vi "FPGA Main.vi"() -> ()   [LabVIEW 2017]
doc: "This VI will continually read single point values from 4 channels of an analog input module at a specified rate."
uses:
  <vilib>/LabVIEW Targets/FPGA/cRIO/shared/nicrio_ModuleControls/nicrio_cRIO-9205_VoltageRange.ctl
  <vilib>/LabVIEW Targets/FPGA/cRIO/shared/nicrio_ModuleControls/nicrio_cRIO-9205_TerminalMode.ctl
  <vilib>/rvi/Emulation/niFpgaGetClockAttributes.vi
  <vilib>/rvi/Emulation/niFpgaSctlEmulationGetInTimedLoop.vi
  <vilib>/rvi/Emulation/niFpgaEmulationReportErrorSimple.vi
  Instance           1 31Saved   NI 9203 Basic IO (FPGA) .vi
  <vilib>/rvi/eio/common/nirviEmuTemplateMethod_errors.vi
  <vilib>/rvi/interface/RandomDataEmulation/niFpgaRandomDataHandleErrors.vi
  <vilib>/rvi/Emulation/niFpgaCriticalErrorInLSC.vi
  <vilib>/eio/EIOMethodNode/EIOMethodNode.xnode
  <vilib>/eio/EIONode/EIONode.xnode
  <vilib>/rvi/DataTransferAndStorage/Container/XNode/niFpgaContainer.xnode
  <vilib>/rvi/interface/RandomDataEmulation/nirviRandomDataFpgaReadWriteTemplate.vi
panel:
  in  "AI Channel Settings":T3(array[cluster])=[{"Voltage Range"=enum."+/- 10V", "Terminal Mode"=enum."RSE"}, {"Voltage Range"=enum."+/- 10V", "Terminal Mode"=enum."RSE"}, {"Voltage Range"=enum."+/- 10V", "Terminal Mode"=enum."RSE"}, {"Voltage Range"=enum."+/- 10V", "Terminal Mode"=enum."RSE"}]
  out "Data FIFO Full":bool
  out "FPGA Error Out":errorcluster
  in  "Update AI Settings":bool
  in  "Loop Rate (uS)":u32
  in  "Stop":bool
  # "For instructions, and select Help>>Show Context Help and hover over the icon."
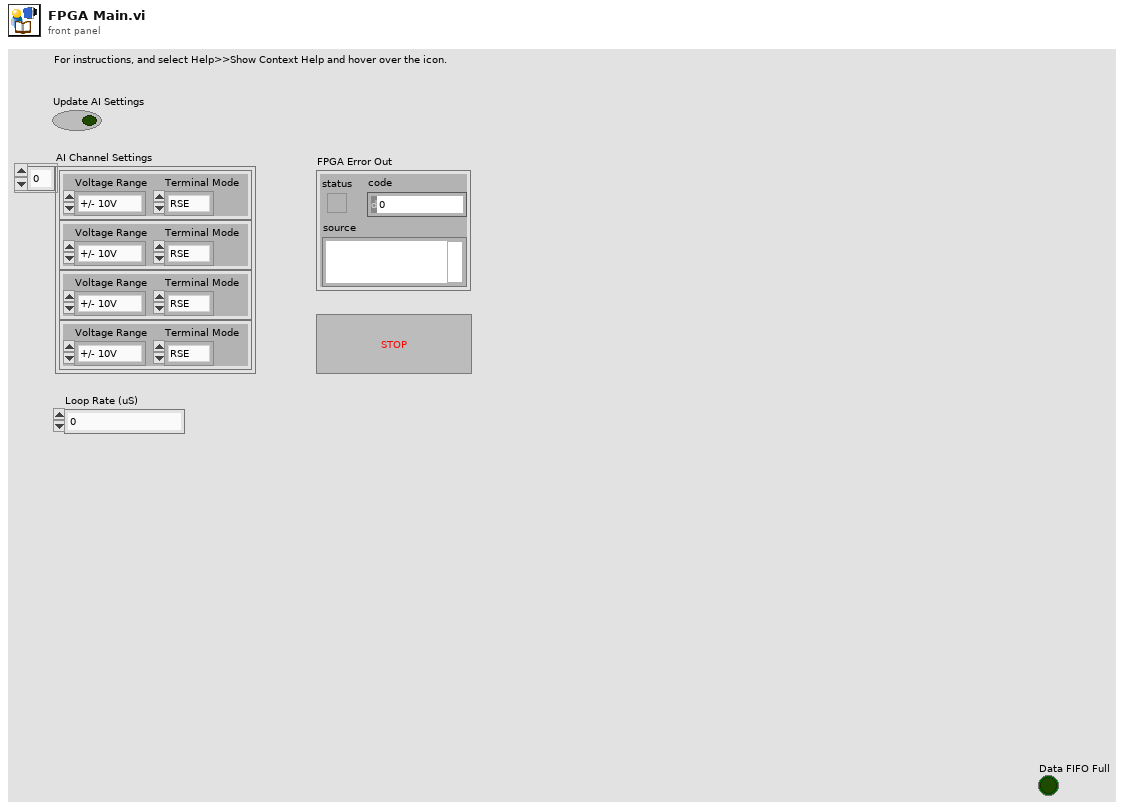
[diagram p1: front panel]
types:
  T1 = typedef "nicrio_cRIO-9205_VoltageRange.ctl" = enum8{"+/- 10V", "+/- 5V", "+/- 1V", "+/- 200mV"}
  T2 = typedef "nicrio_cRIO-9205_TerminalMode.ctl" = enum8{"RSE", "NRSE", "DIFF"}
  T3 = cluster{"Voltage Range":T1, "Terminal Mode":T2}[]
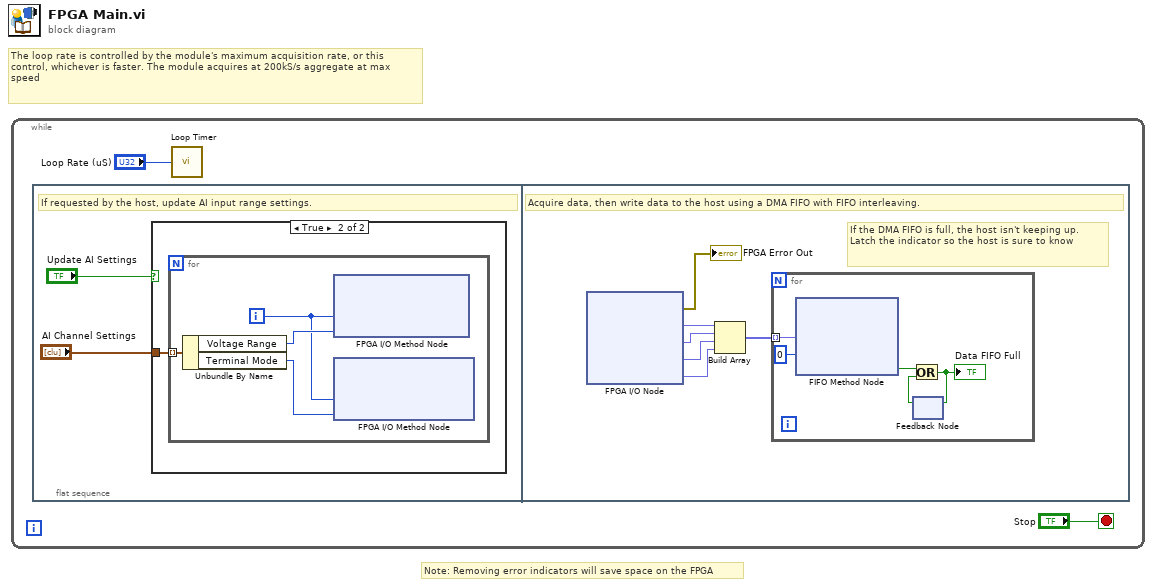
[diagram p0: block diagram]
diagram:
  # "Note: Removing error indicators will save space on the FPGA"
  # "The loop rate is controlled by the module's maximum acquisition rate, or this control, whichever is faster. The module acquires at 200kS/s aggregate at max speed"
  n1 = while {
    stop <- "Stop" stop-if-true
    n2 = flat-sequence {
      frame #0 {
        # "If requested by the host, update AI input range settings."
        n3 = case shown="True" "Update AI Settings" {
          tunnel: "AI Channel Settings" -> [_ w5]
          frame False {
          }
          frame True {
            n4 = for {
              tunnel: w5 -> [w9] mode=indexing
              i -> [w6]
              n5 = Unbundle By Name(w9) -> ("Voltage Range"=w7:T1, "Terminal Mode"=w8:T2)
              n6 = xnode "FPGA I/O Method Node"("AI Channel"=w6, "Voltage Range"=w7) -> ()  [unwired: 1 in, 1 out]
              n7 = xnode "FPGA I/O Method Node"("AI Channel"=w6, "Terminal Mode"=w8) -> ()  [unwired: 1 in, 1 out]
            }
          }
        }
      }
      frame #1 {
        # "If the DMA FIFO is full, the host isn't keeping up. \nLatch the indicator so the host is sure to know"
        # "Acquire data, then write data to the host using a DMA FIFO with FIFO interleaving."
        n8 = xnode "FPGA I/O Node"() -> ("error out"=→"FPGA Error Out":errorcluster, "Mod2/AI0"=w14:fxp<+/-,26,5>, "Mod2/AI1"=w12:fxp<+/-,26,5>, "Mod2/AI2"=w11:fxp<+/-,26,5>, "Mod2/AI3"=w10:fxp<+/-,26,5>)  [unwired: 5 in, 4 out]
        n9 = Build Array(w14, w12, w11, w10) -> (w15:fxp<+/-,26,5>[])
        n10 = for {
          tunnel: w15 -> [w20] mode=indexing
          n11 = xnode ("FIFO Method Node")("Element"=w20, "Timeout"=0) -> ("Timed Out?"=w16:bool)  [unwired: 1 in, 1 out]
          n12 = feedback #1() -> (w18:bool)  [unwired: 1 out]
          n13 = Or(x=w16, y=w18) -> (x .or. y?=w17:bool)
          "Data FIFO Full" <- w17
          n14 = feedback-in #1(w17) -> ()
        }
      }
    }
    n15 = call "Loop Timer"("Count(uSec)"="Loop Rate (uS)") -> ()  [unwired: 1 out]
  }
